vi "FHPP.vi"(7 "Cyle (ms)":i32=50, 8 "error in (no error)":errorcluster, 10 "Use FCT":bool, 11 "IP Address":string="10.0.3.6") -> (0 "error out":errorcluster, 3 "FHPP out":refnum<class "FHPP.lvclass">)   [LabVIEW 2022 SP3, in "FHPP.lvclass"]
uses:
  FHPP.lvclass
  TypeDefs/CCON.ctl
  TypeDefs/Operating Mode.ctl
  TypeDefs/CPOS.ctl
  TypeDefs/SCON.ctl
  TypeDefs/SPOS.ctl
  TypeDefs/FCT Request.ctl
  TypeDefs/ReqID.ctl
  TypeDefs/FCT Response.ctl
  TypeDefs/ResID.ctl
  TypeDefs/DIR.ctl
  TypeDefs/Setpoints.ctl
  FHPP.lvclass/FHPP.ctl
  <vilib>/Modbus/master/Create Master Instance (TCP).vi
  Loop.vi
  <vilib>/Modbus/master/Modbus Master.lvclass
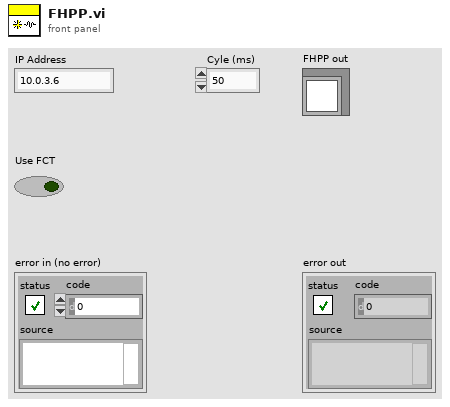
[diagram p1: front panel]
types:
  T1 = typedef "FHPP.lvclass/Setpoints.ctl" = cluster{"Vel/VelRamp (%)":u8, "Setpoint":u32}
  T2 = typedef "FHPP.lvclass/DIR.ctl" = cluster{"Relative":bool, "Control Mode":enum8{"Position", "Force", "Velocity", "Reserved"}, "Function":enum8{"Reserved", "External Input", "External Input with  Cam", "Virtual Master with Cam"}, "Function Group":enum8{"No Function", "Reserver 1", "Reserved 2", "Reserved 3"}, "Camming":bool}
  T3 = typedef "FHPP.lvclass/FCT Response.ctl" = cluster{"ResID":T4, "PNU":u16, "Subindex":u16, "Data":u32}
  T4 = typedef "FHPP.lvclass/ResID.ctl" = u8
  T5 = typedef "FHPP.lvclass/FCT Request.ctl" = cluster{"Request":T6, "PNU":u16, "Subindex":u16, "Data":u32}
  T6 = typedef "FHPP.lvclass/ReqID.ctl" = u8
  T7 = typedef "FHPP.lvclass/SPOS.ctl" = cluster{"Halt":bool, "Ack Start":bool, "Motion Complete":bool, "Ack Teach":bool, "Axis Moving":bool, "Drag Error":bool, "Standstill Control":bool, "Axis Referenced":bool}
  T8 = typedef "FHPP.lvclass/SCON.ctl" = cluster{"Drive Enabled":bool, "Operation Enabled":bool, "Warning":bool, "Error":bool, "Load Voltage Applied":bool, "FCT/MMI":bool, "Operation Mode":T9}
  T9 = typedef "FHPP.lvclass/Operating Mode.ctl" = enum16{"Record Selection", "Direct Mode", "Reserved 1", "Reserved 2"}
  T10 = typedef "FHPP.lvclass/CPOS.ctl" = cluster{"Halt":bool, "Start":bool, "Start Homing":bool, "Jog Positive":bool, "Jog Negative":bool, "Teach Actual Value":bool, "Clear Remaining Pos":bool, "Reserved":bool}
  T11 = typedef "FHPP.lvclass/CCON.ctl" = cluster{"Enabled Drive":bool, "Stop":bool, "Open Brake":bool, "Reset Fault":bool, "Reserved":bool, "Lock Software Access":bool, "Operating Mode":T9}
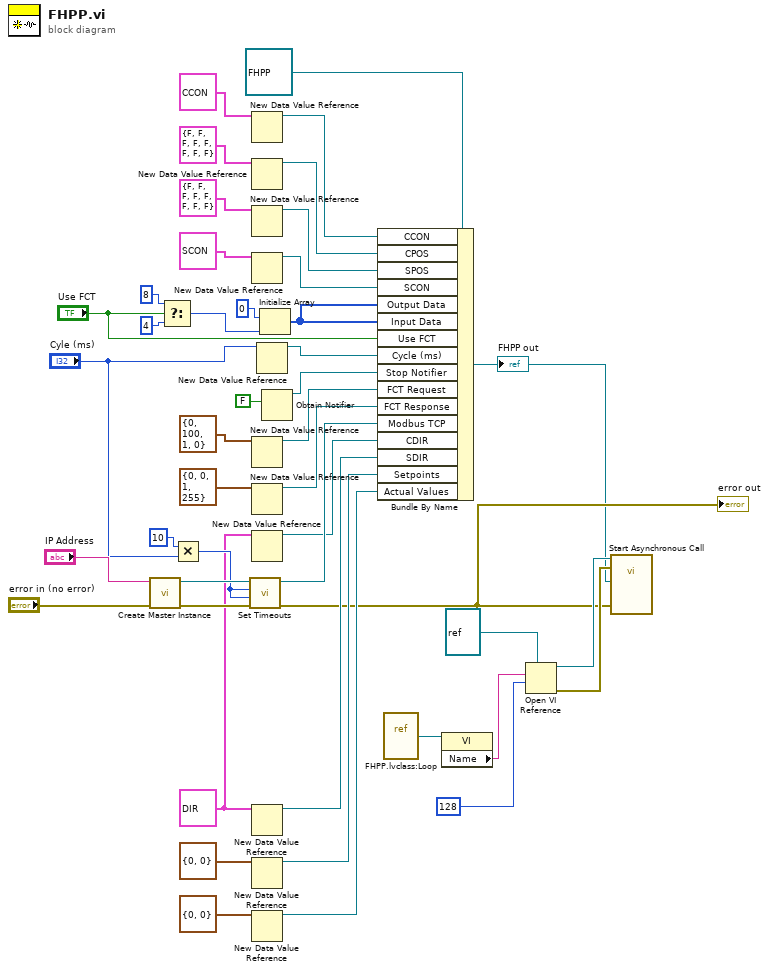
[diagram p0: block diagram]
diagram:
  w14 = T2 {"Relative"=FALSE, "Control Mode"=enum."Position", "Function"=enum."Reserved", "Function Group"=enum."No Function", "Camming"=FALSE} ("DIR")
  n1 = call-poly <vilib>:"Create Master Instance.vi"("error in (no error)"="error in (no error)", "address"="IP Address") -> ("error out"=w20:errorcluster, "TCP master instance"=w21:refnum<class "Modbus Master.lvclass">)  [unwired: 8 in]
  n2 = Select(t=8 ("dimension size"), s="Use FCT", f=4 ("dimension size")) -> (s? t:f=w29:i32)
  n3 = Multiply(x=10 ("y"), y="Cyle (ms)") -> (x*y=w18:i32)
  n4 = call <vilib>:"Set Timeouts.vi"("error in (no error)"=w20, "write operation timeout (ms)"=w18, "read operation timeout (ms)"=w18, "Modbus master in"=w21) -> ("error out"=w2:errorcluster, "Modbus master out"=w17:refnum<class "Modbus Master.lvclass">)  [unwired: 6 in]
  "error out" <- w2
  n5 = New Data Value Reference(data value=T11 {"Enabled Drive"=FALSE, "Stop"=FALSE, "Open Brake"=FALSE, "Reset Fault"=FALSE, "Reserved"=FALSE, "Lock Software Access"=FALSE, "Operating Mode"=enum."Record Selection"} ("CCON")) -> (data value reference=w40:refnum<data-value>)  [unwired: 1 in, 1 out]
  n6 = New Data Value Reference(data value=T10 {"Halt"=FALSE, "Start"=FALSE, "Start Homing"=FALSE, "Jog Positive"=FALSE, "Jog Negative"=FALSE, "Teach Actual Value"=FALSE, "Clear Remaining Pos"=FALSE, "Reserved"=FALSE} ("CPOS")) -> (data value reference=w35:refnum<data-value>)  [unwired: 1 in, 1 out]
  n7 = New Data Value Reference(data value=T7 {"Halt"=FALSE, "Ack Start"=FALSE, "Motion Complete"=FALSE, "Ack Teach"=FALSE, "Axis Moving"=FALSE, "Drag Error"=FALSE, "Standstill Control"=FALSE, "Axis Referenced"=FALSE} ("SPOS")) -> (data value reference=w36:refnum<data-value>)  [unwired: 1 in, 1 out]
  n8 = New Data Value Reference(data value=T8 {"Drive Enabled"=FALSE, "Operation Enabled"=FALSE, "Warning"=TRUE, "Error"=TRUE, "Load Voltage Applied"=FALSE, "FCT/MMI"=FALSE, "Operation Mode"=enum."Record Selection"} ("SCON")) -> (data value reference=w38:refnum<data-value>)  [unwired: 1 in, 1 out]
  n9 = New Data Value Reference(data value=T5 {"Request"=0, "PNU"=100, "Subindex"=1, "Data"=0} ("FCT Request")) -> (data value reference=w26:refnum<data-value>)  [unwired: 1 in, 1 out]
  n10 = New Data Value Reference(data value=T3 {"ResID"=0, "PNU"=0, "Subindex"=1, "Data"=255} ("FCT Response")) -> (data value reference=w25:refnum<data-value>)  [unwired: 1 in, 1 out]
  n11 = New Data Value Reference(data value=w14) -> (data value reference=w15:refnum<data-value>)  [unwired: 1 in, 1 out]
  n12 = New Data Value Reference(data value=w14) -> (data value reference=w13:refnum<data-value>)  [unwired: 1 in, 1 out]
  n13 = New Data Value Reference(data value=T1 {"Vel/VelRamp (%)"=0, "Setpoint"=0} ("Setpoints")) -> (data value reference=w11:refnum<data-value>)  [unwired: 1 in, 1 out]
  n14 = New Data Value Reference(data value=T1 {"Vel/VelRamp (%)"=0, "Setpoint"=0} ("Setpoints")) -> (data value reference=w9:refnum<data-value>)  [unwired: 1 in, 1 out]
  n15 = New Data Value Reference(data value="Cyle (ms)") -> (data value reference=w22:refnum<data-value>)  [unwired: 1 in, 1 out]
  n16 = Initialize Array(u16 0 ("element"), w29) -> (w42:u16[])
  n17 = Obtain Notifier(notification data type=FALSE) -> (notifier out=w27:refnum<notifier>)  [unwired: 3 in, 2 out]
  n18 = Bundle By Name(cluster=refnum<class "FHPP.lvclass"> refnum ("FHPP out"), "CCON"=w40, "CPOS"=w35, "SPOS"=w36, "SCON"=w38, "Output Data"=w42, "Input Data"=w42, "Use FCT"="Use FCT", "Cycle (ms)"=w22, "Stop Notifier"=w27, "FCT Request"=w26, "FCT Response"=w25, "Modbus TCP"=w17, "CDIR"=w15, "SDIR"=w13, "Setpoints"=w11, "Actual Values"=w9) -> (w1:refnum<class "FHPP.lvclass">)
  "FHPP out" <- w1
  n19 = vi-ref "FHPP.lvclass:Loop.vi"() -> (w7:refnum<vi>)
  n20 = property class="VI"(reference=w7) -> ("Name"=w6:string)  [unwired: 1 in, 2 out]
  n21 = Open VI Reference(type specifier VI Refnum (for type only)=refnum<vi> refnum, vi path=w6, options=128) -> (vi reference=w5:refnum<vi>, error out=w3:errorcluster)  [unwired: 3 in]
  n22 = call-by-ref "Start Asynchronous Call"(reference=w5, error in=w3, 8:"error in (no error)"=w2, "FHPP in"=w1) -> ()  [unwired: 8 in, 4 out]
